vi "Untitled 9.vi"() -> ()   [LabVIEW 2013]
uses:
  <vilib>/myRIO/Instrument Drivers/Onboard IO/Encoder/vis/Smart Open.vi
  <vilib>/myRIO/Instrument Drivers/Onboard IO/Encoder/vis/Read.vi
  <vilib>/myRIO/Instrument Drivers/Onboard IO/PWM/vis/Smart Open.vi
  <vilib>/myRIO/Instrument Drivers/Onboard IO/PWM/vis/Set Duty Cycle and Frequency.vi
  <vilib>/myRIO/Instrument Drivers/Onboard IO/DIO/vis/Smart Open.vi
  <vilib>/myRIO/Instrument Drivers/Onboard IO/DIO/vis/Write.vi
  <vilib>/myRIO/Instrument Drivers/Onboard IO/Encoder/vis/Open.vi
  <vilib>/myRIO/Instrument Drivers/Onboard IO/PWM/vis/Open.vi
  <vilib>/myRIO/Instrument Drivers/Onboard IO/DIO/vis/Open.vi
  <vilib>/Utility/error.llb/Error Cluster From Error Code.vi
  <vilib>/addons/control/pid/pid.llb/PID (DBL).vi
  <vilib>/addons/control/pid/pid.llb/PID Control Input Filter (DBL).vi
  <vilib>/imath/engines/lvmath2/RunTimeEngine/NodeEndStatement/NIMS_NodeEndStatement_Output.vi
  <instcachedir>/0/NIMS_NodeEndStatement_Output_53EC0D466D134D7ABD903AC30B43404B.lvgen/NIMS_NodeEndStatement_Output_53EC0D466D134D7ABD903AC30B43404B_001.vi
  <vilib>/imath/engines/lvmath2/RunTimeEngine/ErrorHandling/NIMS_Finalize Error.vi
  <vilib>/addons/control/pid/NI_PID_pid.lvlib
panel:
  in  "pwm freq":dbl=550.0
  in  "min_out":dbl=33.0
  out "theta_e_sp (rad)":dbl format="%.2f"
  out "XY Graph":cluster{i32[], dbl[]}[](graph)
  out "Boolean":bool
  out "position (m)":dbl
  in  "Reset  theta":bool
  in  "Reset position":bool
  in  "Start controller":bool
  in  "Enable Motor Motor":bool
  out "theta_e (rad)":dbl
  in  "Position Control Gain":T1={"proportional gain (Kc)"=1.0, "integral time (Ti, min)"=0.01, "derivative time (Td, min)"=0.0} {"derivative time (Td, min)" format="%.3f"; "integral time (Ti, min)" format="%.3f"; "proportional gain (Kc)" format="%.3f"}
  in  "position sp (m)":dbl format="%.2f"
  in  "Pendulum Stabilization Gain":T1={"proportional gain (Kc)"=1.0, "integral time (Ti, min)"=0.01, "derivative time (Td, min)"=0.0} {"derivative time (Td, min)" step=1e-05 format="%.5f"; "integral time (Ti, min)" format="%.3f"; "proportional gain (Kc)" format="%.3f"}
  in  "theta_e_offset":dbl
  in  "stop":bool
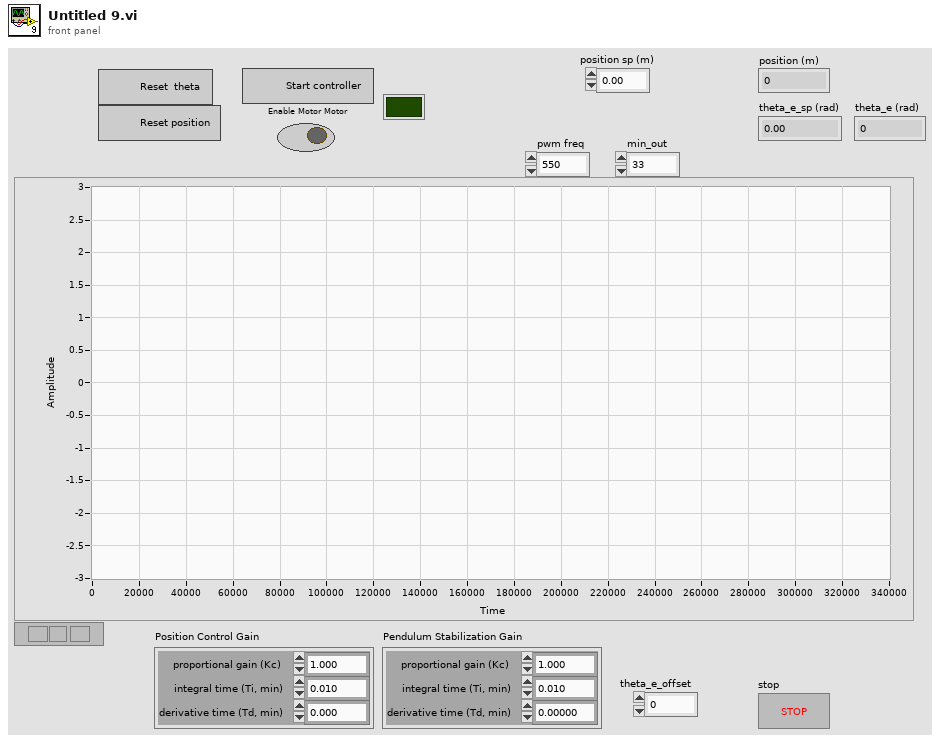
[diagram p1: front panel]
types:
  T1 = cluster{"proportional gain (Kc)":dbl, "integral time (Ti, min)":dbl, "derivative time (Td, min)":dbl}
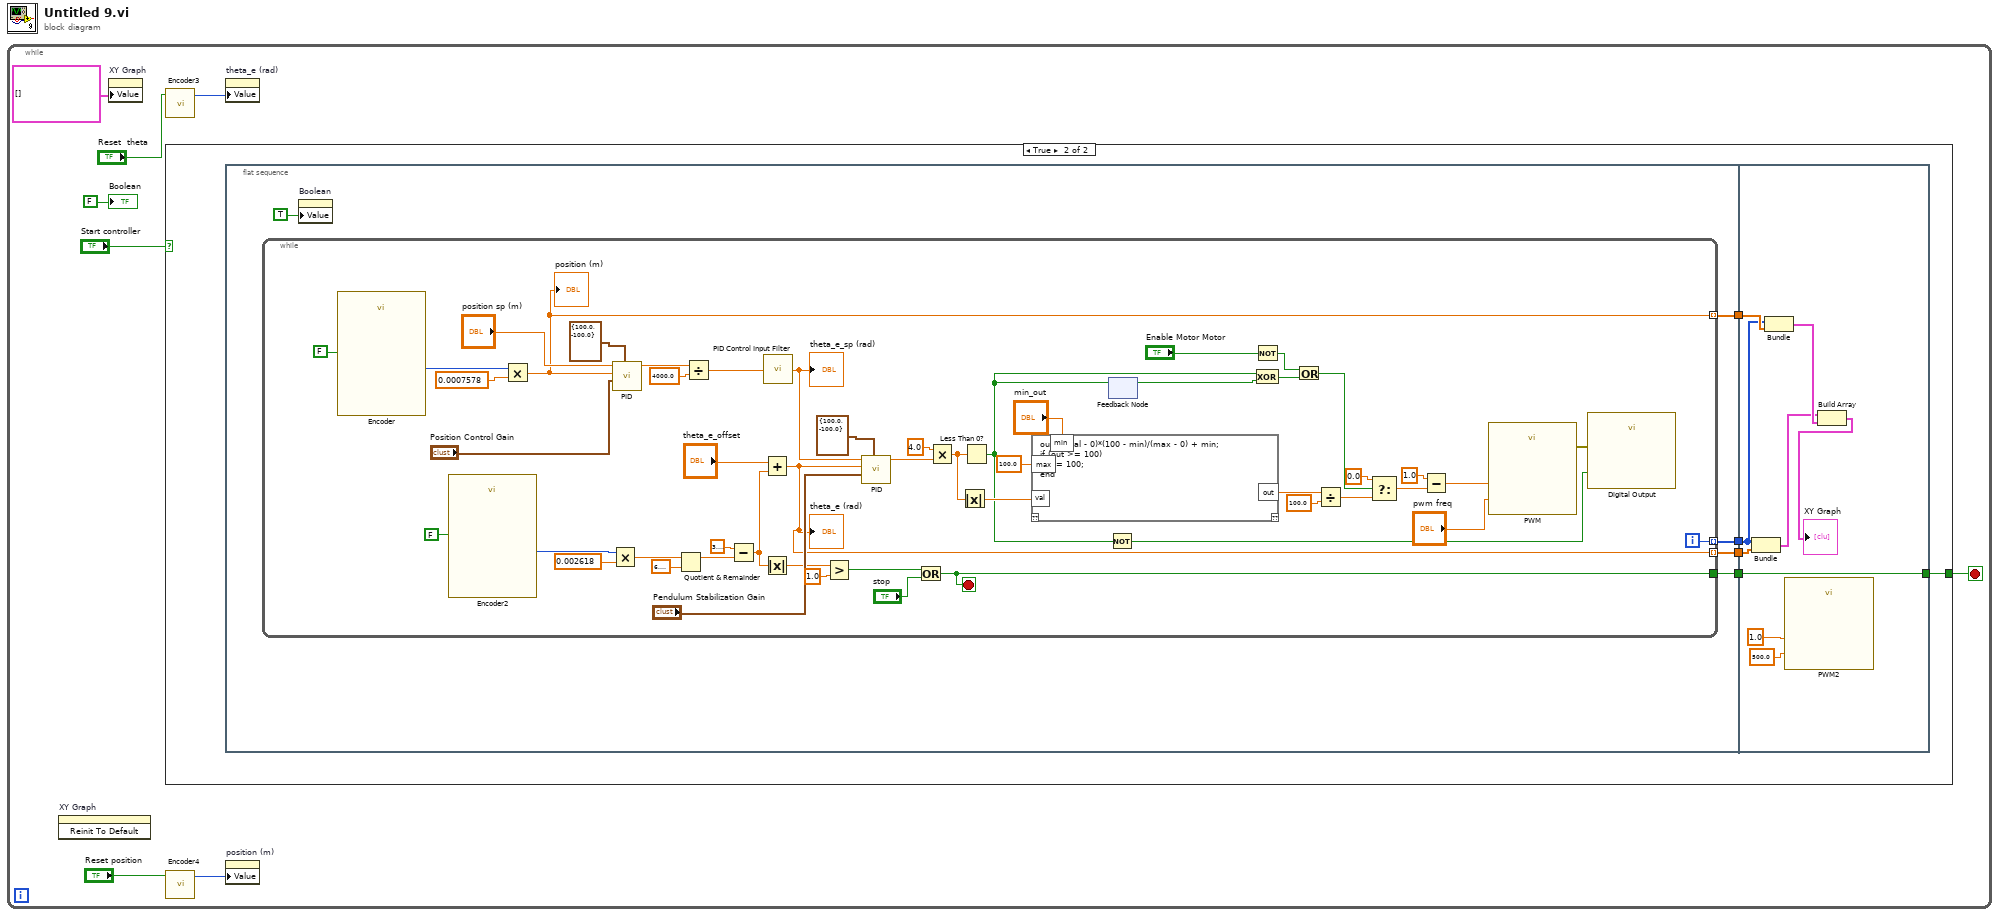
[diagram p0: block diagram]
diagram:
  n1 = while {
    stop <- w8 stop-if-true
    n2 = invoke on="XY Graph" class="XYGraph (strict)" method="Reinit To Default"() -> ()  [unwired: 3 in, 3 out]
    n3 = property on="XY Graph" class="XYGraph (strict)"("Value"=cluster{i32[], dbl[]}[] [] ("XY Graph")) -> ()  [unwired: 2 in, 2 out]
    n4 = call "Encoder3"("Reset Counter"="Reset  theta") -> ("Counter Value"=w4:i32)  [unwired: 23 in, 3 out]
    n5 = case shown="True" "Start controller" {
      tunnel: [_ w13] -> w8
      frame False {
      }
      frame True {
        n6 = flat-sequence {
          tunnel: [w18] -> w12
          tunnel: [w16] -> w11
          tunnel: [w15] -> w10
          tunnel: [w14] -> w9
          tunnel: [w126] -> w13
          tunnel: w12 -> [w126]
          tunnel: w11 -> [w121]
          tunnel: w10 -> [w123]
          tunnel: w9 -> [w122]
          frame #0 {
            n7 = while {
              tunnel: [w28] -> w18
              tunnel: [w22] -> w16 mode=indexing
              tunnel: [w19] -> w15 mode=indexing
              tunnel: [w21] -> w14 mode=indexing
              i -> [w22]
              stop <- w28 stop-if-true
              n8 = call "Encoder"("Reset Counter"=FALSE ("Reset Counter 2")) -> ("Counter Value"=w45:i32)  [unwired: 23 in, 3 out]
              n9 = call "Encoder2"("Reset Counter"=FALSE) -> ("Counter Value"=w48:i32)  [unwired: 23 in, 3 out]
              n10 = Multiply(x=w45, y=0.0007578 ("y 2")) -> (x*y=w21:dbl)
              "position (m)" <- w21
              n11 = Multiply ("Multiply 3")(x=w48, y=0.002618 ("y 3")) -> (x*y=w49:dbl)
              n12 = call-poly <vilib>:"PID.vi"("output range"=cluster{"output high":dbl, "output low":dbl} {"output high"=100.0, "output low"=-100.0}, "PID gains"="Position Control Gain", "process variable"=w21, "setpoint"="position sp (m)") -> ("output"=w27:dbl)  [unwired: 6 in, 1 out]
              n13 = Quotient & Remainder(x=w49, y=6.283185307179586 ("Constant 2")) -> (x-y*floor(x/y)=w42:dbl)  [unwired: 1 out]
              n14 = Divide(x=w27, y=4000.0 ("x")) -> (x/y=w25:dbl)
              n15 = Subtract(x=3.141592653589793, y=w42) -> (x-y=w20:dbl)
              n16 = Add(x="theta_e_offset", y=w20) -> (x+y=w19:dbl)
              "theta_e (rad)" <- w19
              n17 = Absolute Value(x=w20) -> (abs(x)=w33:dbl)
              n18 = call-poly <vilib>:"PID Control Input Filter.vi"("input"=w25) -> ("output"=w24:dbl)  [unwired: 4 in]
              "theta_e_sp (rad)" <- w24
              n19 = Greater?(x=w33, y=1.0) -> (0:w30:bool)
              n20 = call-poly <vilib>:"PID.vi"("output range"=cluster{"output high":dbl, "output low":dbl} {"output high"=100.0, "output low"=-100.0}, "PID gains"="Pendulum Stabilization Gain", "process variable"=w19, "setpoint"=w24) -> ("output"=w36:dbl)  [unwired: 6 in, 1 out]
              n21 = Or(x=w30, y="stop") -> (x .or. y?=w28:bool)
              n22 = Multiply(x=4.0, y=w36) -> (x*y=w35:dbl)
              n23 = Absolute Value ("Absolute Value 2")(x=w35) -> (abs(x)=w58:dbl)
              n24 = Less Than 0?(x=w35) -> (x < 0?=w52:bool)
              n25 = mathscript code="out = (val - 0)*(100 - min)/(max - 0) + min;\nif (out >= 100)\nout = 100;\nend"("val"=w58, "max"=100.0 ("max_in"), "min"="min_out") -> ("out"=w56:dbl)  [unwired: 1 in, 1 out]
              n26 = Not ("Not 2")(x=w52) -> (.not. x?=w23:bool)
              n27 = feedback #1 ("Feedback Node 2")() -> (w61:bool)  [unwired: 1 in]
              n28 = feedback-in #1 ("3")(w52) -> ()
              n29 = Not(x="Enable Motor Motor") -> (.not. x?=w64:bool)
              n30 = Exclusive Or(1:w61, 2:w52) -> (0:w65:bool)
              n31 = Or ("Or 2")(x=w64, y=w65) -> (x .or. y?=w62:bool)
              n32 = Divide(x=w56, y=100.0 ("y 3")) -> (x/y=w54:dbl)
              n33 = Select(t=0.0, s=w62, f=w54) -> (s? t:f=w66:dbl)
              n34 = Subtract(x=1.0, y=w66) -> (x-y=w59:dbl)
              n35 = call "PWM"("Duty Cycle (0-1)"=w59, "Frequency (Hz)"="pwm freq") -> ("error out"=w69:errorcluster)  [unwired: 25 in]
              n36 = call "Digital Output"("A/DIO6 (Pin 23)"=w23, "error in (no error)"=w69) -> ()  [unwired: 25 in, 1 out]
            }
            n37 = property on="Boolean" class="Bool (strict)"("Value"=TRUE ("Boolean")) -> ()  [unwired: 2 in, 2 out]
          }
          frame #1 {
            n38 = Bundle(w121, w123) -> (w119:cluster{i32[], dbl[]})  [unwired: 1 in]
            n39 = Bundle(w121, w122) -> (w120:cluster{i32[], dbl[]})  [unwired: 1 in]
            n40 = call "PWM2"("Duty Cycle (0-1)"=1.0, "Frequency (Hz)"=500.0) -> ()  [unwired: 25 in, 1 out]
            n41 = Build Array(w119, w120) -> (→"XY Graph":cluster{i32[], dbl[]}[])
          }
        }
      }
    }
    n42 = call "Encoder4"("Reset Counter"="Reset position") -> ("Counter Value"=w3:i32)  [unwired: 23 in, 3 out]
    n43 = property on="theta_e (rad)" class="DigNum (strict)"("Value"=w4) -> ()  [unwired: 2 in, 2 out]
    n44 = property on="position (m)" class="DigNum (strict)"("Value"=w3) -> ()  [unwired: 2 in, 2 out]
    "Boolean" <- FALSE
  }
